vi "Init.vi"(8 "error in (no error)":errorcluster, 11 "SECSGEM in":refnum<class "SECSGEM.lvclass">) -> (0 "error out":errorcluster, 3 "SECSGEM out":refnum<class "SECSGEM.lvclass">)   [LabVIEW 2022 SP3, in "SECSGEM.lvclass"]
uses:
  SECSGEM.lvclass
  SECSGEM.lvclass/SECSGEM.ctl
  C:/Users/Josh.Thibeault/Desktop/SecsPort.dll
  Users/Josh.Thibeault/Desktop/SecsPort.dll
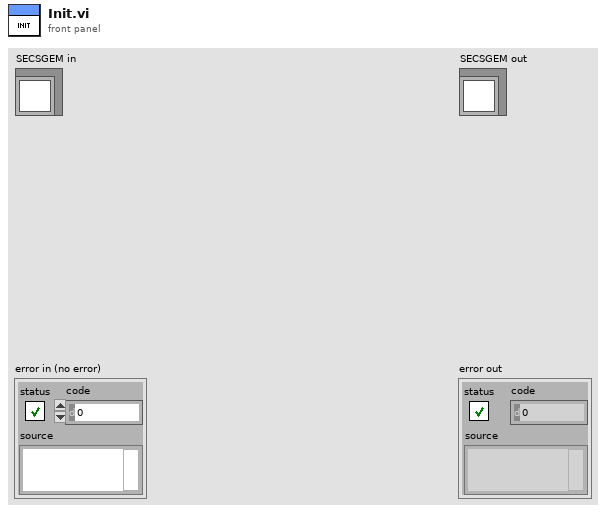
[diagram p1: front panel]
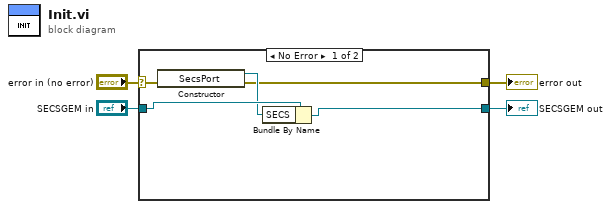
[diagram p0: block diagram]
diagram:
  n1 = case shown="No Error" "error in (no error)" {
    selector: "error in (no error)" -> [w6 w11]
    tunnel: [w5 w11] -> w3
    tunnel: [w8 w10] -> w1
    tunnel: "SECSGEM in" -> [w9 w10]
    frame No Error {
      n2 = constructor class="SecsPort"(error in=w6) -> (reference out=w7:refnum<k24>, error out=w5:errorcluster)  [unwired: 2 in, 1 out]
      n3 = Bundle By Name(cluster=w9, "SECS"=w7) -> (w8:refnum<class "SECSGEM.lvclass">)
    }
    frame Error {
    }
  }
  "error out" <- w3
  "SECSGEM out" <- w1
